vi "createStreamingDataAlgorithm.vi"(8 "error in (no error)":errorcluster, 10 "Stream Mode Algorithm":T1, 11 "ISDAFactory in":refnum<class "ISDAFactory.lvclass">) -> (0 "error out":errorcluster, 2 "StreamingDataAlgorithm":refnum<class "StreamingDataAlgorithm.lvclass">, 3 "ISDAFactory out":refnum<class "ISDAFactory.lvclass">)   [LabVIEW 2013, in "ISDAFactory.lvclass"]
uses:
  ISDAFactory.lvclass
  StreamingDataAlgorithm/StreamingDataAlgorithm.lvclass
  Configuration/Stream Mode Algorithm.ctl
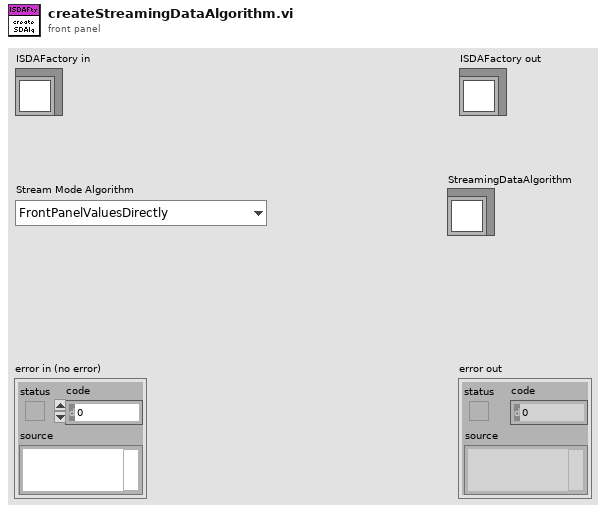
[diagram p1: front panel]
types:
  T1 = typedef "Stream Mode Algorithm.ctl" = enum16{"FrontPanelValuesDirectly"}
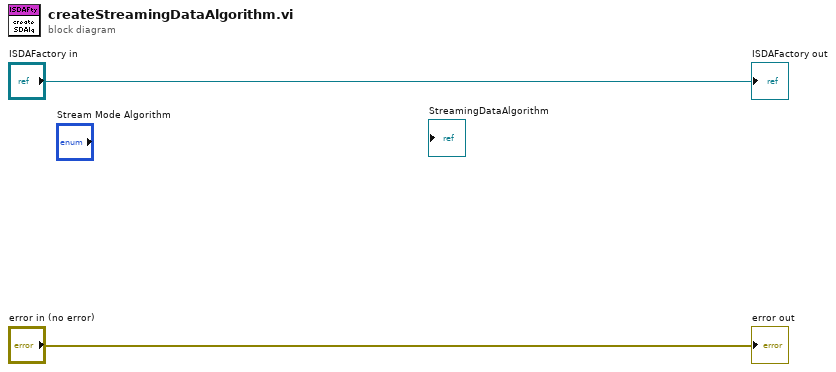
[diagram p0: block diagram]
diagram:
  "error out" <- "error in (no error)"
  "ISDAFactory out" <- "ISDAFactory in"
